vi "Get Current Date and Time.vi"() -> (3 "Date and time string":string)   [LabVIEW 2024]
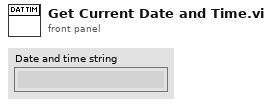
[diagram p1: front panel]
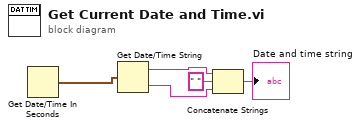
[diagram p0: block diagram]
diagram:
  n1 = Get Date/Time In Seconds() -> (seconds since 1Jan1904=w5:timestamp)
  n2 = Get Date/Time String(seconds (now)=w5) -> (date string=w3:string, time string=w2:string)  [unwired: 2 in]
  n3 = Concatenate Strings(w3, " " ("string"), w2) -> (→"Date and time string":string)
